vi "_Report Strings.vi"(8 "error in":errorcluster, 10 "data in":T1(array[cluster]), 11 "vi name in":string) -> (0 "error out":errorcluster, 2 "test jsons out":string[](array[string]), 3 "ats jsons out":string[](array[string]))   [LabVIEW 2022 SP3]
uses:
  Arcadia/Common/Framework/ATS Composite Output.ctl
  Arcadia/Common/Framework/ATS Test Output.ctl
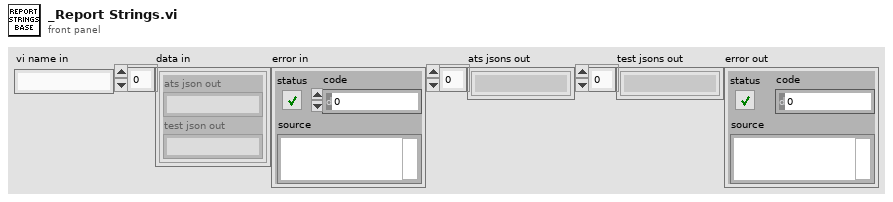
[diagram p1: front panel]
types:
  T1 = cluster{"ats json out":string, "test json out":string}[]
  T2 = typedef "ATS Composite Output.ctl" = cluster{"Test Case Jsons":cluster{"ats json":string, "test json":string}[], "Schema Version":u32, "Schema Oldest Compatible Version":u32}
  T3 = typedef "ATS Test Output.ctl" = cluster{"Test Case":string, "Pass":bool, "Skipped":bool, "Skip Reason":string, "Test Error":errorcluster, "Start Timestamp":string, "Test Time (s)":dbl, "Custom Target Name":string, "Use Custom Device List":bool, "Custom Device List":string[], "Cancel Retry":bool, "Schema Version":u32, "Schema Oldest Compatible Version":u32}
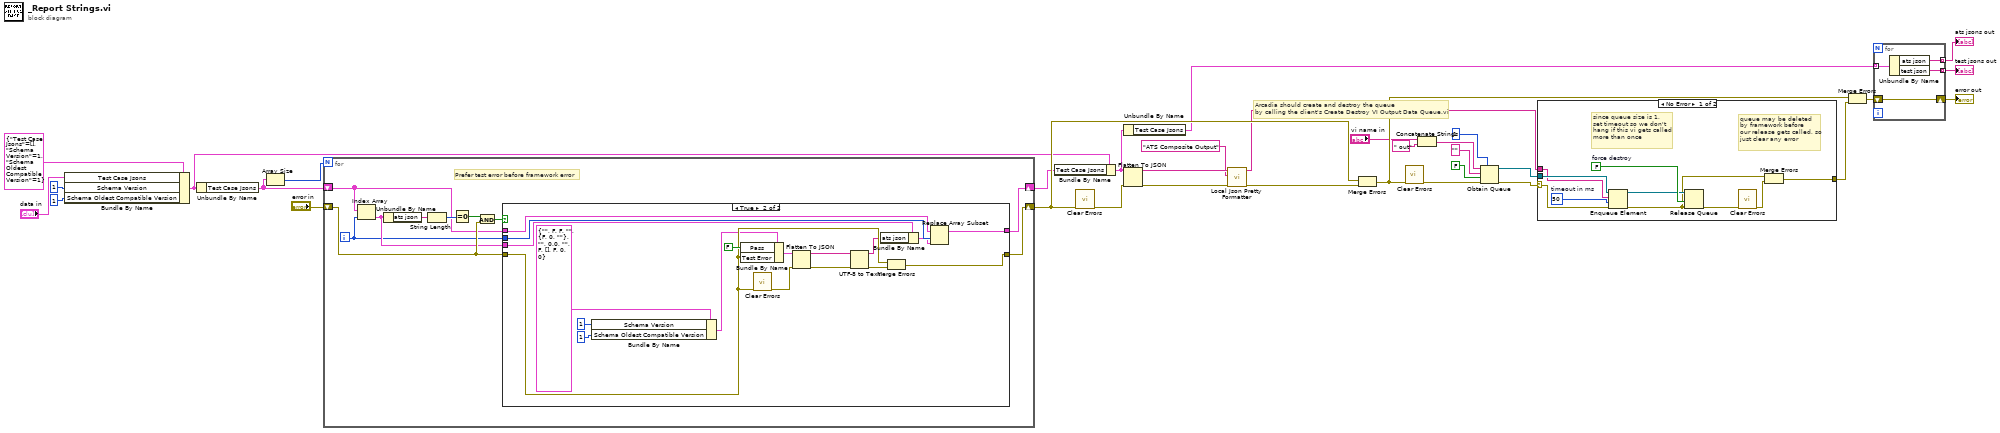
[diagram p0: block diagram]
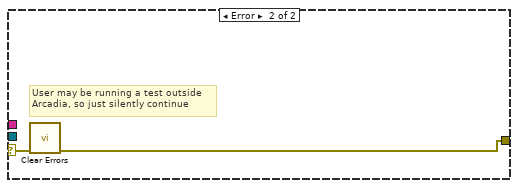
[diagram p3: hidden frame]
diagram:
  # "Arcadia should create and destroy the queue\nby calling the client's Create Destroy VI Output Data Queue.vi"
  n1 = Bundle By Name(cluster=T2 {"Test Case Jsons"=[], "Schema Version"=1, "Schema Oldest Compatible Version"=1} ("ATS Composite Output"), "Test Case Jsons"="data in", "Schema Version"=u32 1, "Schema Oldest Compatible Version"=u32 1) -> (w15:T2)
  n2 = Unbundle By Name(w15) -> ("Test Case Jsons"=w6:cluster{"ats json":string, "test json":string}[])
  n3 = Array Size(array=w6) -> (size(s)=w5:i32)
  n4 = for {
    N: w5 -> [_]
    shift-right: [w39] -> w20
    shift-left: "error in" -> [w40]
    shift-right: [w35] -> w12
    shift-left: w6 -> [w36]
    i -> [w34]
    # "Prefer test error before framework error"
    n5 = Index Array(array=w36, index=w34) -> (element=w37:cluster{"ats json":string, "test json":string})
    n6 = Unbundle By Name(w37) -> ("ats json"=w38:string)
    n7 = String Length(string=w38) -> (length=w43:i32)
    n8 = Equal To 0?(x=w43) -> (x = 0?=w42:bool)
    n9 = And(x=w42, y=w40) -> (x .and. y?=w41:bool)
    n10 = case shown="True" w41 {
      tunnel: [w45 w62] -> w39
      tunnel: w40 -> [w45 w59]
      tunnel: w37 -> [_ w50]
      tunnel: w36 -> [w44 w49]
      tunnel: [w44 w48] -> w35
      tunnel: w34 -> [_ w47]
      frame False {
      }
      frame True {
        n11 = Bundle By Name(cluster=T3 {"Test Case"="", "Pass"=FALSE, "Skipped"=FALSE, "Skip Reason"="", "Test Error"={"status"=FALSE, "code"=0, "source"=""}, "Start Timestamp"="", "Test Time (s)"=0.0, "Custom Target Name"="", "Use Custom Device List"=FALSE, "Custom Device List"=[], "Cancel Retry"=FALSE, "Schema Version"=0, "Schema Oldest Compatible Version"=0} ("ATS Test Output"), "Schema Version"=u32 1, "Schema Oldest Compatible Version"=u32 1) -> (w57:T3)
        n12 = Bundle By Name(cluster=w57, "Pass"=FALSE, "Test Error"=w59) -> (w58:T3)
        n13 = call <vilib>:"Clear Errors.vi"("error in (no error)"=w59) -> ("error out"=w63:errorcluster)  [unwired: 5 in, 1 out]
        n14 = Flatten To JSON(anything=w58, error in (no error)=w63) -> (JSON string=w52:string, 11:w54:errorcluster)  [unwired: 1 in]
        n15 = UTF-8 to Text(8:w54, 11:w52) -> (0:w53:errorcluster, 3:w51:string)  [unwired: 1 in]
        n16 = Bundle By Name(cluster=w50, "ats json"=w51) -> (w46:cluster{"ats json":string, "test json":string})
        n17 = Merge Errors(w59, w53) -> (w62:errorcluster)
        n18 = Replace Array Subset "Replace Array Subset"(array=w49, new element=w46, index=w47) -> (w48:cluster{"ats json":string, "test json":string}[])
      }
    }
  }
  n19 = Bundle By Name(cluster=w15, "Test Case Jsons"=w12) -> (w11:T2)
  n20 = call <vilib>:"Clear Errors.vi"("error in (no error)"=w20) -> ("error out"=w22:errorcluster)  [unwired: 5 in, 1 out]
  n21 = Unbundle By Name(w11) -> ("Test Case Jsons"=w10:cluster{"ats json":string, "test json":string}[])
  n22 = Flatten To JSON(anything=w11, error in (no error)=w22) -> (JSON string=w29:string, 11:w27:errorcluster)  [unwired: 1 in]
  n23 = call "Local Json Pretty Formatter.vi"("error in"=w27, "data name in"="ATS Composite Output" ("data name"), "json in"=w29) -> ("error out"=w23:errorcluster, "json out"=w19:string)  [unwired: 7 in]
  n24 = Merge Errors(w20, w23) -> (w21:errorcluster)
  n25 = call <vilib>:"Clear Errors.vi"("error in (no error)"=w21) -> ("error out"=w25:errorcluster)  [unwired: 5 in, 1 out]
  n26 = Concatenate Strings("vi name in", " out" ("string")) -> (w13:string)
  n27 = Obtain Queue(max queue size (-1, unlimited)=1, name (unnamed)=w13, element data type="", create if not found? (T)=FALSE, error in (no error)=w25) -> (queue out=w31:refnum<queue>, error out=w24:errorcluster)  [unwired: 1 out]
  n28 = case shown="No Error" w24 {
    selector: w24 -> [w68 w75]
    tunnel: [w66 w74] -> w33
    tunnel: w31 -> [w72 _]
    tunnel: w19 -> [w69 _]
    frame No Error {
      w64 = 50  # timeout in ms
      w71 = FALSE  # force destroy
      # "since queue size is 1,\nset timeout so we don't\nhang if this vi gets called\nmore than once"
      # "queue may be deleted\nby framework before \nour release gets called, so\njust clear any error"
      n29 = Enqueue Element(queue=w72, element=w69, timeout in ms (-1)=w64, error in (no error)=w68) -> (queue out=w70:refnum<queue>, error out=w65:errorcluster)  [unwired: 1 out]
      n30 = Release Queue(queue=w70, force destroy? (F)=w71, error in (no error)=w65) -> (error out=w73:errorcluster)  [unwired: 2 out]
      n31 = call <vilib>:"Clear Errors.vi"("error in (no error)"=w73) -> ("error out"=w67:errorcluster)  [unwired: 5 in, 1 out]
      n32 = Merge Errors(w65, w67) -> (w66:errorcluster)
    }
    frame Error {
      # "User may be running a test outside\nArcadia, so just silently continue"
      n33 = call <vilib>:"Clear Errors.vi"("error in (no error)"=w75) -> ("error out"=w74:errorcluster)  [unwired: 5 in, 1 out]
    }
  }
  n34 = Merge Errors(w21, w33) -> (w3:errorcluster)
  n35 = for {
    tunnel: w10 -> [w79] mode=indexing
    tunnel: [w78] -> w8 mode=indexing
    tunnel: [w77] -> w9 mode=indexing
    shift-right: [w76] -> w4
    shift-left: w3 -> [w76]
    n36 = Unbundle By Name(w79) -> ("ats json"=w78:string, "test json"=w77:string)
  }
  "error out" <- w4
  "ats jsons out" <- w8
  "test jsons out" <- w9
